vi "waaka_tare.vi"(8 "Update":bool, 11 "Input weight":dbl) -> (2 "Output weight":dbl)   [LabVIEW 2016]
panel:
  in  "Offset weight":dbl
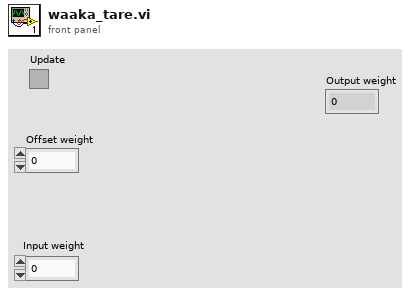
[diagram p1: front panel]
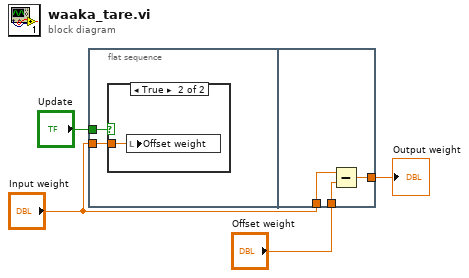
[diagram p0: block diagram]
diagram:
  n1 = flat-sequence {
    tunnel: "Input weight" -> [w6]
    tunnel: "Update" -> [w5]
    tunnel: "Input weight" -> [w10]
    tunnel: "Offset weight" -> [w9]
    tunnel: [w8] -> w1
    frame #0 {
      n2 = case shown="True" w5 {
        tunnel: w6 -> [_ w7]
        frame False {
        }
        frame True {
          n3 = local write "Offset weight"(w7) -> ()
        }
      }
    }
    frame #1 {
      n4 = Subtract(x=w10, y=w9) -> (x-y=w8:dbl)
    }
  }
  "Output weight" <- w1
